vi "NIVS Public Docs Path.vi"() -> (3 "NI VeriStand publid docs path":path)   [LabVIEW 2013, in "Project Wizard.lvlib"]
uses:
  <vilib>/Utility/sysdir.llb/System Directory Type.ctl
  Project Wizard.lvlib
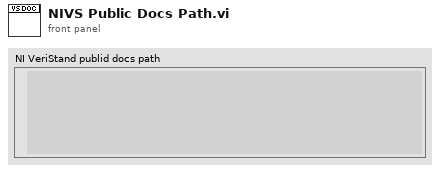
[diagram p1: front panel]
types:
  T1 = typedef "System Directory Type.ctl" = i32
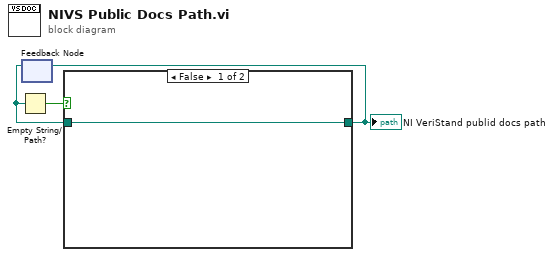
[diagram p0: block diagram]
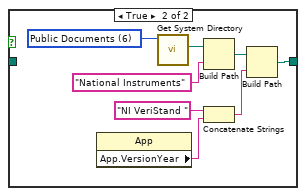
[diagram p2: hidden frame]
diagram:
  n1 = feedback #1() -> (w1:path)  [unwired: 1 in]
  n2 = Empty String/Path?(string/path=w1) -> (empty?=w2:bool)
  n3 = case shown="False" w2 {
    tunnel: [w4 w7] -> w3
    tunnel: w1 -> [w4 _]
    frame False {
    }
    frame True {
      w12 = T1 6 items=["User Home"=0, "User Desktop"=1, "User Documents"=2, "User Application Data"=3, "User Preferences"=4, "User Temporary"=5, "Public Documents"=6, "Public Application Data"=7, "Public Preferences"=8, "Public Cache"=13, "System Core Libraries"=9, "System Installed Libraries"=10, "Application Files"=11, "Boot Volume Root"=12] ("system directory type")
      n4 = property class="App"() -> ("App.VersionYear"=w10:string)  [unwired: 2 in, 2 out]
      n5 = call <vilib>:"Get System Directory.vi"("system directory type"=w12) -> ("system directory"=w11:path)  [unwired: 10 in]
      n6 = Build Path(base path=w11, name or relative path="National Instruments") -> (appended path=w6:path)
      n7 = Concatenate Strings("NI VeriStand " ("string"), w10) -> (w8:string)
      n8 = Build Path(base path=w6, name or relative path=w8) -> (appended path=w7:path)
    }
  }
  "NI VeriStand publid docs path" <- w3
  n9 = feedback-in #1(w3) -> ()
